vi "Get Control Data.vi"(8 "error in (no error)":errorcluster, 11 "Panel":refnum<vi>) -> (0 "error out":errorcluster, 1 "Control Data":T1[](array[typedef]), 2 "Indicators":string[][](array[string]), 3 "Controls":string[][](array[string]))   [LabVIEW 2023, in "VI Properties Editor.lvlib"]
uses:
  VI Properties Editor.lvlib
  Control Properties.ctl
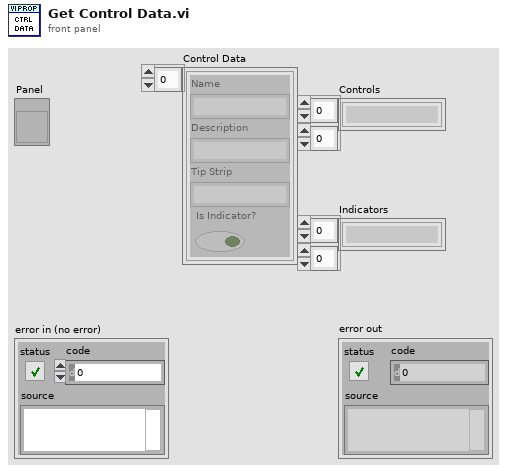
[diagram p1: front panel]
types:
  T1 = typedef "VI Properties Editor.lvlib/Control Properties.ctl" = cluster{"Name":string, "Description":string, "Tip Strip":string, "Is Indicator?":bool}
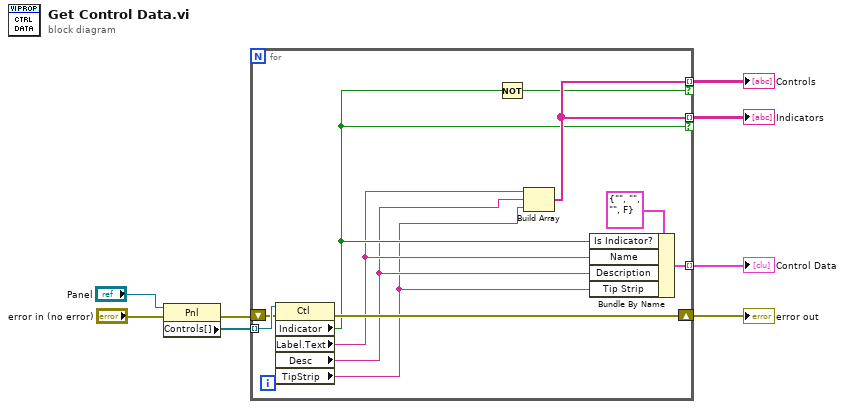
[diagram p0: block diagram]
diagram:
  n1 = property class="Pnl"(reference="Panel", error in="error in (no error)") -> (error out=w8:errorcluster, "Controls[]"=w7:refnum<vi>[])  [unwired: 1 out]
  n2 = for {
    tunnel: w7 -> [w18] mode=indexing
    shift-right: [w19] -> w6
    shift-left: w8 -> [w17]
    tunnel: [w16] -> w3 mode=indexing if=w14
    tunnel: [w16] -> w2 mode=indexing if=w13
    tunnel: [w9] -> w1 mode=indexing
    n3 = property class="Ctl"(reference=w18, error in=w17) -> (error out=w19:errorcluster, "Indicator"=w13:bool, "Label.Text"=w12:string, "Desc"=w11:string, "TipStrip"=w10:string)  [unwired: 1 out]
    n4 = Not(x=w13) -> (.not. x?=w14:bool)
    n5 = Build Array(w12, w11, w10) -> (w16:string[])
    n6 = Bundle By Name(cluster=T1 {"Name"="", "Description"="", "Tip Strip"="", "Is Indicator?"=FALSE} ("Control Properties"), "Is Indicator?"=w13, "Name"=w12, "Description"=w11, "Tip Strip"=w10) -> (w9:T1)
  }
  "error out" <- w6
  "Controls" <- w3
  "Indicators" <- w2
  "Control Data" <- w1
